vi "for_v0_v32.vi"() -> ()   [LabVIEW 2009]
panel:
  in  "h":dbl(slide)=87.56476683937824 scale=0.0..100.0
  in  "d":dbl(knob)=6.8275981187706005 scale=0.0..10.0
  in  "v":dbl(slide)=2.6550522648083623 scale=3.0..0.0
  out "Iteratia":dbl=7.0
  in  "stop":bool
  out "Picture":picture
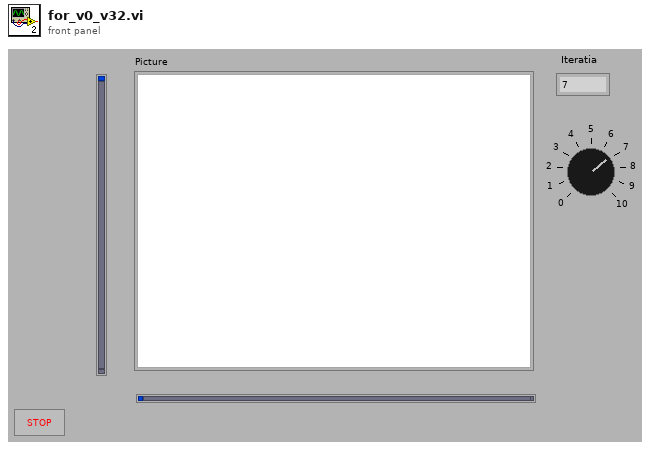
[diagram p1: front panel]
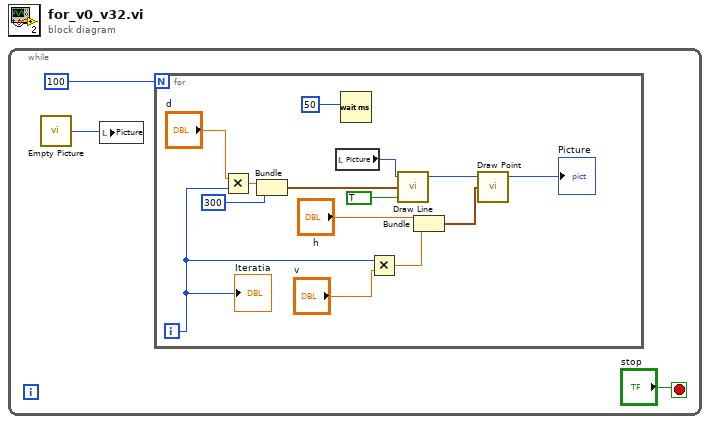
[diagram p0: block diagram]
diagram:
  n1 = while {
    stop <- "stop" stop-if-true
    n2 = call "Empty Picture"() -> ("empty picture"=w1:picture)
    n3 = local write "Picture"(w1) -> ()
    n4 = for {
      N: 100 -> [_]
      i -> [w6]
      n5 = Multiply(x="d", y=w6) -> (x*y=w9:dbl)
      n6 = Bundle(w9, 300) -> (w15:cluster{dbl, i32})  [unwired: 1 in]
      n7 = local read "Picture"() -> (w17:picture)
      n8 = Wait (ms)(milliseconds to wait=50) -> ()  [unwired: 1 out]
      n9 = Multiply(x=w6, y="v") -> (x*y=w7:dbl)
      n10 = call <vilib>:"Draw Line.vi"("picture"=w17, "end point"=w15, "absolute coordinates?(T)"=TRUE) -> ("new picture"=w16:picture)  [unwired: 6 in]
      n11 = Bundle("h"="h", w7) -> (w8:cluster{"h":dbl, dbl})  [unwired: 1 in]
      n12 = call <vilib>:"Draw Point.vi"("picture"=w16, "point(x,y)"=w8) -> ("new picture"=→"Picture":picture)  [unwired: 7 in]
      "Iteratia" <- w6
    }
  }
